vi "Write Stage Configuration.vi"(8 "error in (no error)":errorcluster, 10 "Stage Configuration":T1={"Serial Port"="COM3", "Forward Step (mm)"=0.4, "Lane Length (mm)"=6.0, "Lane Separation (mm)"=0.8}, 11 "Stage Controller in":refnum<class "Stage Controller.lvclass">) -> (0 "error out":errorcluster, 3 "Stage Controller out":refnum<class "Stage Controller.lvclass">)   [LabVIEW 2015, in "Stage Controller.lvlib" / "Stage Controller.lvclass"]
uses:
  Stage Controller.lvclass
  Resources/Type Defs/Stage Configuration.ctl
  Stage Controller.lvclass/Stage Controller.ctl
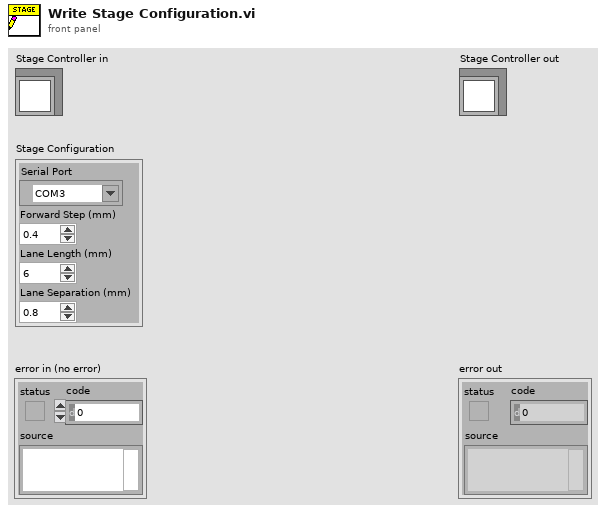
[diagram p1: front panel]
types:
  T1 = typedef "Stage Configuration.ctl" = cluster{"Serial Port":refnum<visa-resource-name>, "Forward Step (mm)":dbl, "Lane Length (mm)":dbl, "Lane Separation (mm)":dbl}
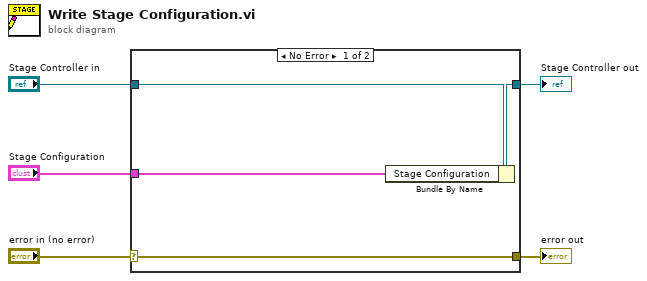
[diagram p0: block diagram]
diagram:
  n1 = case shown="No Error" "error in (no error)" {
    selector: "error in (no error)" -> [w9 w10]
    tunnel: [w9 w10] -> w4
    tunnel: [w7 w11] -> w2
    tunnel: "Stage Controller in" -> [w8 w11]
    tunnel: "Stage Configuration" -> [w6 _]
    frame No Error {
      n2 = Bundle By Name(cluster=w8, "Stage Configuration"=w6) -> (w7:refnum<class "Stage Controller.lvclass">)
    }
    frame Error {
    }
  }
  "error out" <- w4
  "Stage Controller out" <- w2
